vi "test.vi"() -> ()   [LabVIEW 2019]
uses:
  <vilib>/Instr/_visa.llb/VISA Configure Serial Port (Instr).vi
panel:
  out "error out":errorcluster
  in  "stop":bool
  out "RH":dbl
  out "Temp":dbl
  in  "Port":enum8{"ONE", "TWO"}(ring)
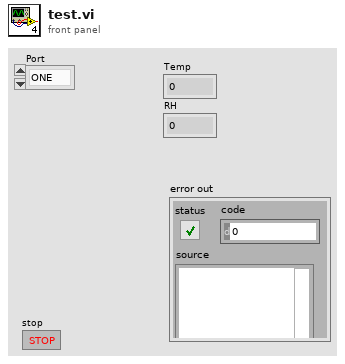
[diagram p1: front panel]
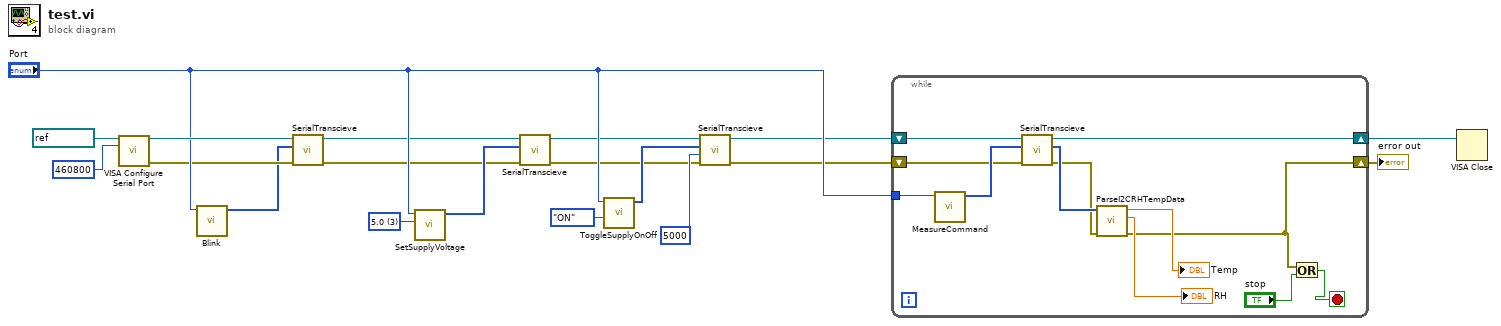
[diagram p0: block diagram]
diagram:
  w14 = u8 3 items=["1.2"=0, "1.5"=4, "1.8"=1, "2.1"=5, "2.4"=6, "2.7"=7, "3,0"=8, "3.3"=2, "3.6"=9, "4.5"=10, "5.0"=3, "5.5"=11] ("Voltage")
  n1 = call-poly "VISA Configure Serial Port"("VISA resource name"=refnum<visa-resource-name> "COM7", "baud rate (9600)"=u32 460800) -> ("VISA resource name out"=w17:refnum<visa-resource-name>, "error out"=w15:errorcluster)  [unwired: 12 in]
  n2 = call "Blink.vi"("Port"="Port") -> ("ByteArrayToSend"=w12:u8[])  [unwired: 10 in]
  n3 = call "SerialTranscieve.vi"("error in (no error)"=w15, "ByteArrayToSend"=w12, "VISA resource name"=w17) -> ("error out"=w4:errorcluster, "VISA resource name out"=w11:refnum<visa-resource-name>)  [unwired: 5 in, 2 out]
  n4 = call "SetSupplyVoltage.vi"("Voltage"=w14, "Port"="Port") -> ("ByteArrayToSend"=w10:u8[])  [unwired: 9 in]
  n5 = call "SerialTranscieve.vi"("error in (no error)"=w4, "ByteArrayToSend"=w10, "VISA resource name"=w11) -> ("error out"=w3:errorcluster, "VISA resource name out"=w9:refnum<visa-resource-name>)  [unwired: 5 in, 2 out]
  n6 = call "ToggleSupplyOnOff.vi"("State"=enum8{"OFF", "ON"}."ON", "Port"="Port") -> ("ByteArrayToSend"=w8:u8[])  [unwired: 9 in]
  n7 = call "SerialTranscieve.vi"("error in (no error)"=w3, "TimeOut(ms)"=u32 5000, "ByteArrayToSend"=w8, "VISA resource name"=w9) -> ("error out"=w2:errorcluster, "VISA resource name out"=w6:refnum<visa-resource-name>)  [unwired: 4 in, 2 out]
  n8 = while {
    tunnel: "Port" -> [w31]
    shift-right: [w28] -> w5
    shift-left: w6 -> [w29]
    shift-right: [w20] -> w1
    shift-left: w2 -> [w25]
    stop <- w21 stop-if-true
    n9 = call "MeasureCommand.vi"("Port"=w31) -> ("ByteArrayToSend"=w27:u8[])  [unwired: 10 in]
    n10 = call "SerialTranscieve.vi"("error in (no error)"=w25, "ByteArrayToSend"=w27, "VISA resource name"=w29) -> ("error out"=w24:errorcluster, "ByteArrayRecieved"=w26:u8[], "VISA resource name out"=w28:refnum<visa-resource-name>)  [unwired: 5 in, 1 out]
    n11 = call "ParseI2CRHTempData.vi"("error in (no error)"=w24, "ByteArrayRecieved"=w26) -> ("error out"=w20:errorcluster, "Numeric"=→"RH":dbl, "Numeric 2"=→"Temp":dbl)  [unwired: 7 in]
    n12 = Or(x=w20, y="stop") -> (x .or. y?=w21:bool)
  }
  "error out" <- w1
  n13 = VISA Close(VISA resource name=w5) -> ()  [unwired: 1 in, 1 out]
